vi "Get Endpoint Configuration.vi"(8 "error in":errorcluster, 10 "endpoint":string, 11 "endpoint configuration in":T2 format="%.0x") -> (0 "error out":errorcluster, 2 "configuration":T1, 3 "endpoint configuration out":T2 format="%.0x")   [LabVIEW 2017, in "SLSC Switch Scripting.lvlib"]
doc: "Returns the configuration for one endpoint."
uses:
  SLSC Switch Scripting.lvlib
  <vilib>/NI Veristand/Custom Device API/Custom Device Item Ref.ctl
  Shared/Endpoint Configuration Enum.ctl
  <vilib>/NI Veristand/Custom Device API/Get Item Property (String).vi
  <vilib>/NI VeriStand/Custom Device API/Custom Device API.lvlib
  Shared/NI-SWITCH Shared.lvlib
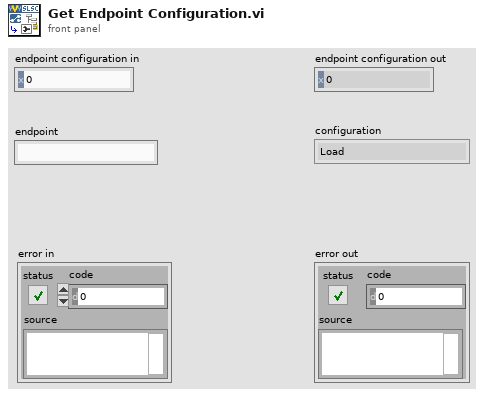
[diagram p1: front panel]
types:
  T1 = typedef "NI-SWITCH Shared.lvlib/Endpoint Configuration Enum.ctl" = enum16{"Load", "Source", "Configuration"}
  T2 = typedef "Custom Device API.lvlib/Custom Device Item Ref.ctl" = u64
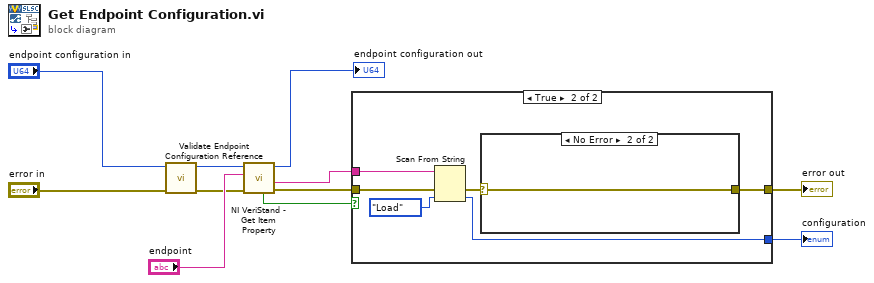
[diagram p0: block diagram]
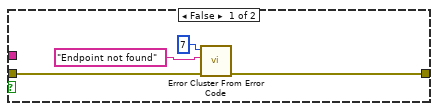
[diagram p2: hidden frame]
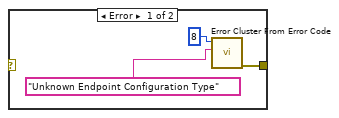
[diagram p3: hidden frame]
diagram:
  n1 = call "Validate Endpoint Configuration Reference.vi"("error in"="error in", "endpoint configuration in"="endpoint configuration in") -> ("error out"=w3:errorcluster, "endpoint configuration out"=w1:T2)  [unwired: 8 in]
  n2 = call-poly <vilib>:"NI VeriStand - Get Item Property.vi"("error in (no error)"=w3, "Property Name"="endpoint", "Item Ref in"=w1) -> ("error out"=w7:errorcluster, "Value"=w6:string, "Item Ref out"=→"endpoint configuration out":T2, "Found?"=w8:bool)  [unwired: 5 in]
  n3 = case shown="True" w8 {
    tunnel: w7 -> [w13 w18]
    tunnel: w6 -> [_ w21]
    tunnel: [_ w20] -> w5
    tunnel: [w12 w17] -> w4
    frame False {
      n4 = call <vilib>:"Error Cluster From Error Code.vi"("error in (no error)"=w13, "error message (\"\")"="Endpoint not found" ("error message (\"\")"), "error code (0)"=7) -> ("error out"=w12:errorcluster)  [unwired: 6 in]
    }
    frame True {
      n5 = Scan From String(input string=w21, error in=w18, default 1=Endpoint_Configuration_Enum."Load" ("Configuration Type")) -> (error out=w16:errorcluster, output 1=w20:T1)  [unwired: 2 in, 2 out]
      n6 = case shown="No Error" w16 {
        selector: w16 -> [_ w25]
        tunnel: [w22 w25] -> w17
        frame Error {
          n7 = call <vilib>:"Error Cluster From Error Code.vi"("error message (\"\")"="Unknown Endpoint Configuration Type" ("error message (\"\")"), "error code (0)"=8) -> ("error out"=w22:errorcluster)  [unwired: 7 in]
        }
        frame No Error {
        }
      }
    }
  }
  "error out" <- w4
  "configuration" <- w5
